vi "start.vi"(8 "error in (no error)":errorcluster, 10 "ILCAppConfig":T1={"ILCConfig"={"Input Channels"=enum."Channel 0", "Scan Rate (Hz) "=enum."50", "ADC PGA Gain"=0}, "RS232Config"={"VISA resource name"="", "Baud Rate"=9600, "Data Bits"=8, "Parity"=enum."None", "Stop Bits"=10, "Flow Control"=0, "Timeout (ms)"=10000}, "Application Timing"={"Loop Period (ms)"=1}} {"Application Timing"."Loop Period (ms)" min=1 max=5000; "RS232Config"."Stop Bits" items=["1.0"=10, "1.5"=15, "2.0"=20]; "RS232Config"."Flow Control" items=["None", "XON/XOFF", "RTS/CTS", "XON/XOFF & RTS/CTS", "DTR/DSR", "XON/XOFF & DTR/DSR"]; "RS232Config"."Data Bits" min=5 max=8 step=1; "ILCConfig"."ADC PGA Gain" max=7}, 11 "Context in":refnum<class "Context.lvclass">) -> (0 "error out":errorcluster, 3 "Context out":refnum<class "Context.lvclass">)   [LabVIEW 2012, in "Context.lvclass"]
uses:
  Context.lvclass
  State/ILCAppConfig.ctl
  Configuration/ILCConfig.ctl
  Configuration/InputChannels.ctl
  Configuration/ScanRate_Hz_MultichannelOptions.ctl
  Configuration/RS232Config.ctl
  Model/Model/ApplicationTiming.ctl
  Context.lvclass/Context.ctl
  State/State.lvclass
  Model/Model/Model.lvclass
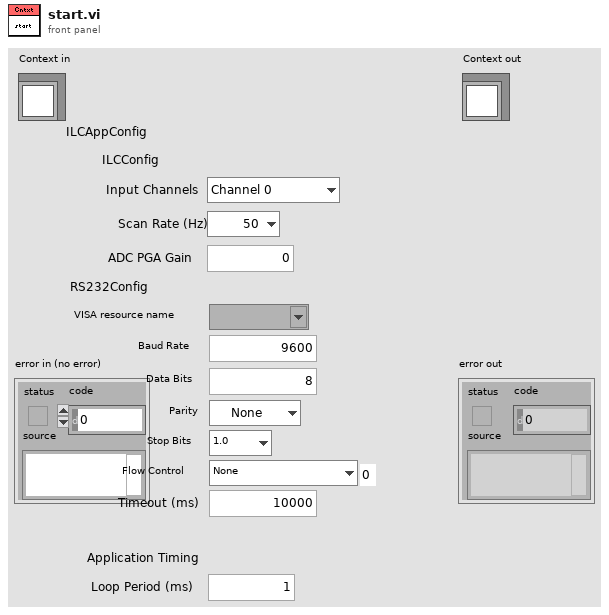
[diagram p1: front panel]
types:
  T1 = typedef "ILCAppConfig.ctl" = cluster{"ILCConfig":T2, "RS232Config":T5, "Application Timing":T6}
  T2 = typedef "ILCConfig.ctl" = cluster{"Input Channels":T3, "Scan Rate (Hz) ":T4, "ADC PGA Gain":u8}
  T3 = typedef "InputChannels.ctl" = enum16{"Channel 0", "3 Channels", "5 Channels"}
  T4 = typedef "ScanRate_Hz_MultichannelOptions.ctl" = enum16{"50", "60", "100", "120", "200", "240", "300", "400", "480", "600", "1200", "2400", "4800"}
  T5 = typedef "RS232Config.ctl" = cluster{"VISA resource name":refnum<visa-resource-name>, "Baud Rate":u32, "Data Bits":u16, "Parity":enum16{"None", "Odd", "Even", "Mark", "Space"}, "Stop Bits":u16, "Flow Control":u16, "Timeout (ms)":u32}
  T6 = typedef "ApplicationTiming.ctl" = cluster{"Loop Period (ms)":u16}
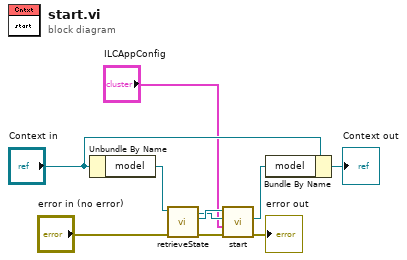
[diagram p0: block diagram]
diagram:
  n1 = Unbundle By Name("Context in") -> ("model"=w9:refnum<class "Model.lvclass">)
  n2 = call "retrieveState.vi"("error in (no error)"="error in (no error)", "Model in"=w9) -> ("error out"=w2:errorcluster, "state"=w10:refnum<class "State.lvclass">, "Model out"=w8:refnum<class "Model.lvclass">)  [unwired: 7 in]
  n3 = call-dynamic "start.vi"("error in (no error)"=w2, "ILCAppConfig"="ILCAppConfig", "model"=w8, "State in"=w10) -> ("error out"=→"error out":errorcluster, "model 2"=w5:refnum<class "Model.lvclass">)  [unwired: 5 in, 1 out]
  n4 = Bundle By Name(cluster="Context in", "model"=w5) -> (→"Context out":refnum<class "Context.lvclass">)
